vi "Controller Get Filter Sets Coefficients.vi"(10 "Filter Set Number":i32, 11 "Filter Sets":dbl[][](array[numeric])) -> (2 "Gains":dbl[][](array[numeric]), 3 "Coefficients":dbl[][](array[numeric]))   [LabVIEW 2011, in "Controller VIs.lvlib"]
uses:
  Controller VIs.lvlib
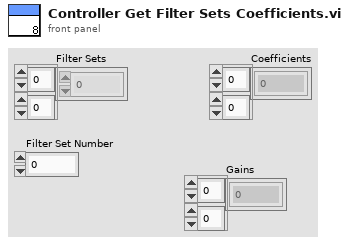
[diagram p1: front panel]
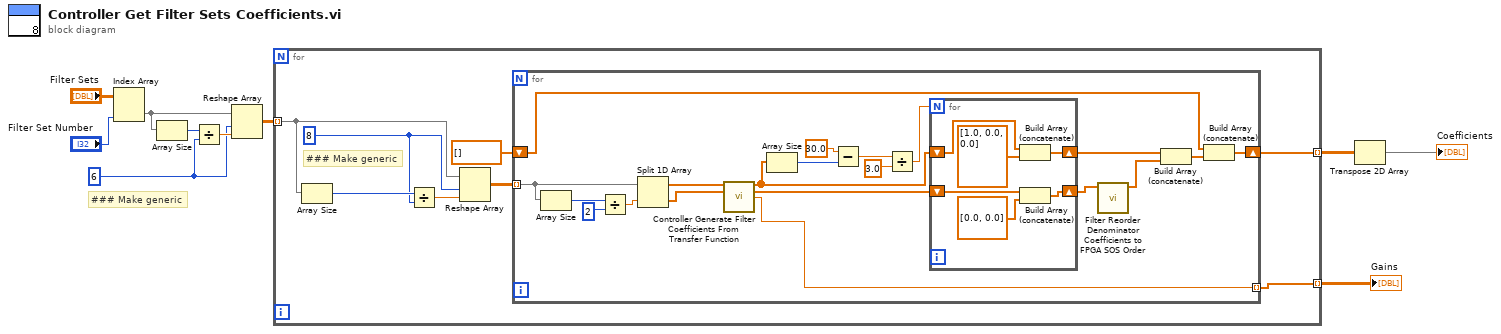
[diagram p0: block diagram]
diagram:
  w4 = 6
  # "### Make generic"
  n1 = Index Array(array="Filter Sets", index (col)="Filter Set Number") -> (element=w8:dbl[])  [unwired: 1 in]
  n2 = Array Size(array=w8) -> (size(s)=w9:i32)
  n3 = Divide(x=w9, y=w4) -> (x/y=w5:dbl)
  n4 = Reshape Array(w8, w4, w5) -> (w6:dbl[][])
  n5 = for {
    tunnel: w6 -> [w16] mode=indexing
    tunnel: [w12] -> w3 mode=indexing
    tunnel: [w11] -> w1 mode=indexing
    w13 = 8
    # "### Make generic"
    n6 = Array Size(array=w16) -> (size(s)=w15:i32)
    n7 = Divide(x=w15, y=w13) -> (x/y=w14:dbl)
    n8 = Reshape Array(w16, w13, w14) -> (w17:dbl[][])
    n9 = for {
      tunnel: w17 -> [w38] mode=indexing
      tunnel: [w21] -> w11 mode=indexing
      shift-right: [w33] -> w12
      shift-left: dbl[] [] -> [w32]
      n10 = Array Size(array=w38) -> (size(s)=w37:i32)
      n11 = Divide(x=w37, y=2) -> (x/y=w35:dbl)
      n12 = Split 1D Array(array=w38, index=w35) -> (first subarray=w23:dbl[], second subarray=w22:dbl[])
      n13 = call "Controller Generate Filter Coefficients From Transfer Function.vi"("numerator"=w23, "denominator"=w22) -> ("coeff b"=w26:dbl[], "coeff a"=w25:dbl[], "gain"=w21:dbl)  [unwired: 11 in]
      n14 = Array Size(array=w26) -> (size(s)=w28:i32)
      n15 = Subtract(x=30.0 ("x*y"), y=w28) -> (x-y=w30:dbl)
      n16 = Divide(x=w30, y=3.0 ("x*y")) -> (x/y=w27:dbl)
      n17 = for {
        N: w27 -> [_]
        shift-right: [w42] -> w24
        shift-left: w26 -> [w44]
        shift-right: [w39] -> w20
        shift-left: w25 -> [w41]
        n18 = Build Array (concatenate)(w44, dbl[] [1.0, 0.0, 0.0]) -> (w42:dbl[])
        n19 = Build Array (concatenate)(w41, dbl[] [0.0, 0.0]) -> (w39:dbl[])
      }
      n20 = call "Filter Reorder Denominator Coefficients to FPGA SOS Order.vi"("coef a (k)"=w20) -> ("coef a (k)"=w19:dbl[])  [unwired: 10 in]
      n21 = Build Array (concatenate)(w24, w19) -> (w34:dbl[])
      n22 = Build Array (concatenate)(w32, w34) -> (w33:dbl[])
    }
  }
  "Gains" <- w1
  n23 = Transpose 2D Array(2D array=w3) -> (transposed array=→"Coefficients":dbl[][])
